vi "mark_check_update.vi"(8 "steps":i32=1000, 9 "mark":i32, 10 "marksArray":T1[](array[typedef]), 11 "Cluster":T4) -> (3 "Boolean":bool)   [LabVIEW 2015, in "PolyVIEW.lvclass"]
uses:
  PolyVIEW.lvclass
  Admin memo.ctl
  actors/world/typedefs/markValue_cluster.ctl
  actors/world/typedefs/markValue.ctl
  actors/world/typedefs/markVolume.ctl
  actors/world/world.lvlib
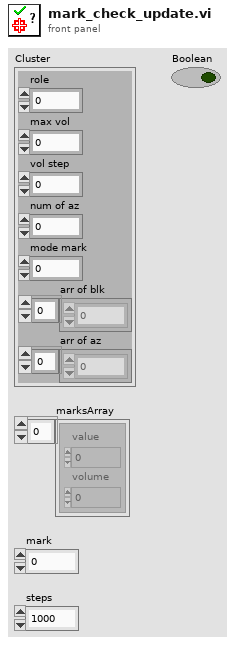
[diagram p1: front panel]
types:
  T1 = typedef "world.lvlib/markValue_cluster.ctl" = cluster{"value":T2, "volume":T3}
  T2 = typedef "world.lvlib/markValue.ctl" = u8
  T3 = typedef "world.lvlib/markVolume.ctl" = u16
  T4 = typedef "PolyVIEW.lvclass/Admin memo.ctl" = cluster{"role":i32, "max vol":i32, "vol step":i32, "num of az":i32, "mode mark":i32, "arr of blk":i32[], "arr of az":i32[]}
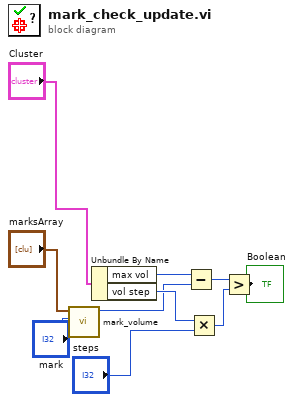
[diagram p0: block diagram]
diagram:
  n1 = call "mark_volume.vi"("element"="mark", "marksArray"="marksArray") -> ("volume"=w3:T3)  [unwired: 9 in]
  n2 = Unbundle By Name("Cluster") -> ("max vol"=w4:i32, "vol step"=w8:i32)
  n3 = Subtract(x=w4, y=w3) -> (x-y=w6:i32)
  n4 = Multiply(x=w8, y="steps") -> (x*y=w7:i32)
  n5 = Greater?(x=w6, y=w7) -> (0:→"Boolean":bool)
